vi "DMM Channel UI.vi"() -> ()   [LabVIEW 2025, in "DMM.lvlib" / "DMM Channel.lvclass"]
doc: "Copyright 2017 National Instruments Corporation\n\nLicensed under the Apache License, Version 2.0 (the \"License\"); you may not use this file except in compliance with the License. You may obtain a copy of the License at http://www.apache.org/licenses/LICENSE-2.0\nUnless required by applicable law or agreed to in writing, software distributed under the License is distributed on an \"AS IS\" BASIS, WITHOUT WARRANTIES OR CONDITIONS OF ANY KIND, either express or implied. See the License for the specific language governing permissions and limitations under the License."
uses:
  DMM Channel.lvclass
  Users/Public/Documents/Sandia National Labs/TSS Plugin/CEF.lvlibp/Node/NodeRef.ctl
  Users/Public/Documents/Sandia National Labs/TSS Plugin/CEF.lvlibp/Node/CEF_Node.lvclass
  Users/Public/Documents/Sandia National Labs/TSS Plugin/CEF.lvlibp/Node/mainQref.ctl
  Users/Public/Documents/Sandia National Labs/TSS Plugin/CEF.lvlibp/Node/UserEventRef.ctl
  Users/Public/Documents/Sandia National Labs/TSS Plugin/Abstract Engine.lvlibp/Plugin/Abstract/Channel configuration/Default Channel.ctl
  C:/Users/Public/Documents/Sandia National Labs/TSS Plugin/CEF.lvlibp/Node/CEF_Node.lvclass
  DMM Channel.lvclass/DMM Channel.ctl
  <vilib>/Utility/error.llb/Trim Whitespace One-Sided.vi
  Users/Public/Documents/Sandia National Labs/TSS Plugin/Abstract Engine.lvlibp/Plugin/Abstract/Channel configuration/Read Channel Setting.vi
  Users/Public/Documents/Sandia National Labs/TSS Plugin/Abstract Engine.lvlibp/Plugin/Abstract/Channel configuration/Write Channel Setting.vi
  Users/Public/Documents/Sandia National Labs/TSS Plugin/Abstract Engine.lvlibp/Plugin/Abstract/Channel configuration/Channel configuration.lvclass
panel:
  in  "Default":T1={"Address"="localhost", "SW Alias"="ch0", "Enabled"=TRUE, "Type"="None", "Description"=""}
  in  "user event":T2
  in  "main queue":T3
  in  "node ref":T4
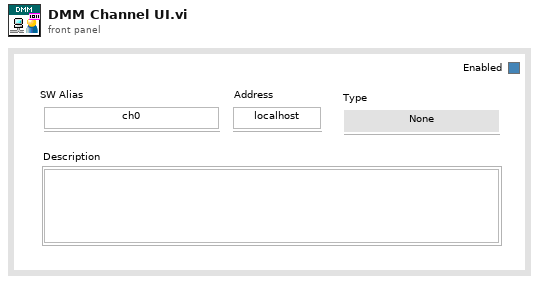
[diagram p1: front panel]
types:
  T1 = typedef "Abstract Engine.lvlibp/Channel configuration.lvclass/Default Channel.ctl" = cluster{"Address":string, "SW Alias":string, "Enabled":bool, "Type":string, "Description":string}
  T2 = typedef "CEF.lvlibp/CEF_Node.lvclass/UserEventRef.ctl" = refnum<user-event>
  T3 = typedef "CEF.lvlibp/CEF_Node.lvclass/mainQref.ctl" = refnum<queue>
  T4 = typedef "CEF.lvlibp/CEF_Node.lvclass/NodeRef.ctl" = refnum<data-value>
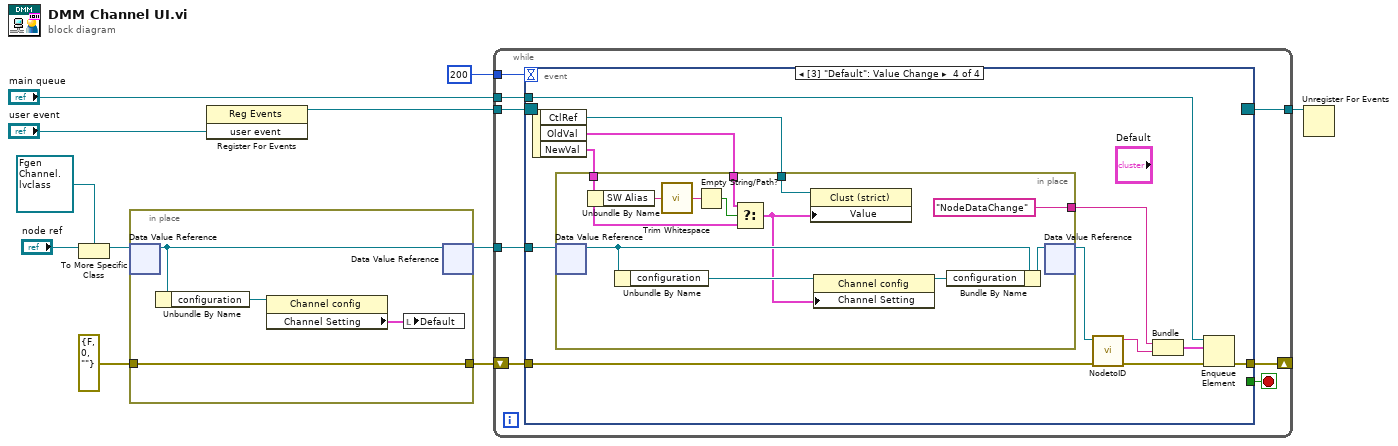
[diagram p0: block diagram]
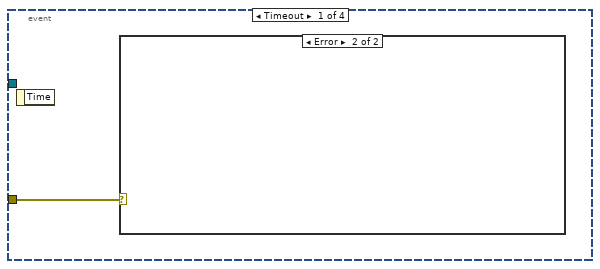
[diagram p2: hidden frame]
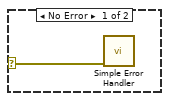
[diagram p3: hidden frame]
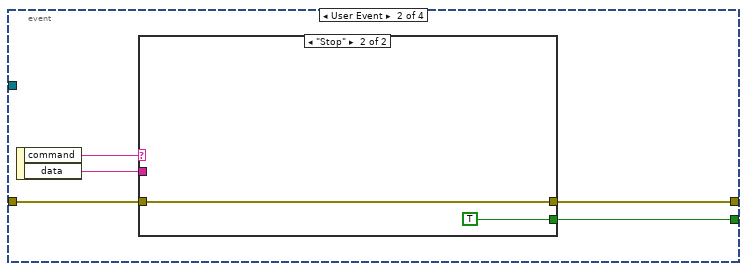
[diagram p4: hidden frame]
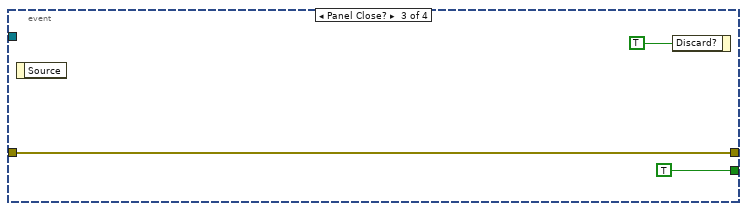
[diagram p6: hidden frame]
diagram:
  n1 = To More Specific Class(target class=refnum<data-value> refnum ("data value reference"), reference="node ref") -> (specific class reference=w2:refnum<data-value>)  [unwired: 1 in, 1 out]
  n2 = in-place {
    in-place-border: errorcluster {"status"=FALSE, "code"=0, "source"=""} ("error out") -> [w13]
    in-place-border: [w13] -> w1
    # "Initialize the front panel controls when loaded"
    n3 = in-place-dvr #1(w2) -> (w14:refnum<class "DMM Channel.lvclass">)  [unwired: 1 out]
    n4 = Unbundle By Name(w14) -> ("configuration"=w15:refnum<class "Channel configuration.lvclass">)
    n5 = property class="Channel config"(reference=w15) -> ("Channel Setting"=w12:T1)  [unwired: 1 in, 2 out]
    n6 = local write "Default"(w12) -> ()
    n7 = in-place-dvr #1(w14) -> (w5:refnum<data-value>)  [unwired: 1 out]
  }
  n8 = register-events("user event") -> (reference out=w10:refnum<event-registration>)  [unwired: 2 in, 1 out]
  n9 = while {
    tunnel: w5 -> [w23]
    tunnel: w10 -> [w22]
    tunnel: [w21] -> w9
    shift-right: [w18] -> _
    shift-left: w1 -> [w20]
    tunnel: "main queue" -> [w17]
    tunnel: 200 -> [w16]
    stop <- w19 stop-if-true
    n10 = event shown="[3] \"Default\": Value Change" {
      selector: w22 -> [_ _ _ _]
      dyn-events: [_ _ _ _] -> w21
      timeout: w16 -> [_ _ _ _]
      tunnel: w23 -> [_ _ _ w46]
      tunnel: [_ w26 w34 w47] -> w18
      tunnel: w20 -> [w24 w27 w34 w39]
      tunnel: [_ w30 TRUE _] -> w19
      tunnel: w17 -> [_ _ _ w48]
      event Timeout {
        n11 = event-data() -> ()  [unwired: 1 in, 1 out]
        n12 = case shown="Error" w24 {
          selector: w24 -> [w25 _]
          frame No Error {
            n13 = call <vilib>:"Simple Error Handler.vi"("error in (no error)"=w25) -> ()  [unwired: 4 in, 5 out]
          }
          frame Error {
          }
        }
      }
      event User Event {
        n14 = event-data() -> ("command"=w28:string, "data"=w29:string)  [unwired: 1 in]
        n15 = case shown="\"Stop\"" w28 {
          tunnel: w29 -> [_ _]
          tunnel: [_ TRUE] -> w30
          tunnel: w27 -> [w31 w32]
          tunnel: [w31 w32] -> w26
          frame Default {
          }
          frame "Stop" {
          }
        }
      }
      event Panel Close? {
        n16 = event-data() -> ()  [unwired: 1 in, 1 out]
        n17 = event-data("Discard?"=TRUE) -> ()  [unwired: 1 in, 1 out]
      }
      event Value Change {
        n18 = event-data() -> ("CtlRef"=w43:refnum<vi>, "OldVal"=w44:T1, "NewVal"=w42:T1)  [unwired: 1 in]
        n19 = in-place {
          in-place-border: w44 -> [w56]
          in-place-border: w42 -> [w53]
          in-place-border: w43 -> [w55]
          in-place-border: ["NodeDataChange" ("Message Name")] -> w41
          n20 = in-place-dvr #2(w46) -> (w60:refnum<class "DMM Channel.lvclass">)  [unwired: 1 out]
          n21 = Unbundle By Name(w53) -> ("SW Alias"=w54:string)
          n22 = Unbundle By Name(w60) -> ("configuration"=w58:refnum<class "Channel configuration.lvclass">)
          n23 = call <vilib>:"Trim Whitespace.vi"("string"=w54) -> ("trimmed string"=w51:string)  [unwired: 1 in]
          n24 = Empty String/Path?(string/path=w51) -> (empty?=w52:bool)
          n25 = Select(t=w56, s=w52, f=w53) -> (s? t:f=w49:T1)
          n26 = property class="Clust (strict)"(reference=w55, "Value"=w49) -> ()  [unwired: 1 in, 2 out]
          n27 = property class="Channel config"(reference=w58, "Channel Setting"=w49) -> (reference out=w57:refnum<class "Channel configuration.lvclass">)  [unwired: 1 in, 1 out]
          n28 = Bundle By Name(cluster=w60, "configuration"=w57) -> (w59:refnum<class "DMM Channel.lvclass">)
          n29 = in-place-dvr #2(w59) -> (w45:refnum<data-value>)  [unwired: 1 out]
        }
        n30 = call "NodetoID.vi"("error in"=w39, "node ref"=w45) -> ("error out"=w38:errorcluster, "ID"=w40:string)  [unwired: 8 in]
        n31 = Bundle("Message Name"=w41, "ID"=w40) -> (w37:cluster{"Message Name":string, "ID":string})  [unwired: 1 in]
        n32 = Enqueue Element(queue=w48, element=w37, error in (no error)=w38) -> (error out=w47:errorcluster)  [unwired: 1 in, 2 out]
      }
    }
  }
  n33 = Unregister For Events(event registration refnum=w9) -> ()  [unwired: 1 in, 1 out]
